vi "ultrasonic.vi"(0 "Ultrasonic configuration":string="{\n  \"type\": \"Ultrasonic\",\n  \"listen_port\": 8900,\n  \"location\": {\n    \"x\": 245.0,\n    \"y\": 0.0,\n    \"z\": 60.0\n  },\n  \"rotation\": {\n    \"pitch\": 0.0,\n    \"yaw\": 0.0,\n    \"roll\": 0.0\n  },\n  \"fc\": 40000.0,\n  \"pwm_factor\": 2.5,\n  \"max_ultrasonic_returns\": 93,\n   \"sbr\": {\n   \"scan_distance\":4.0,\n   \"azimuth_fov\":30.0,\n   \"elevation_fov\": 0.50,\n    \"ray_division_y\": 5.0,\n    \"ray_division_z\": 5.0,\n    \"debug_frustum\": false,\n    \"debug_scan\": false,\n    \"debug_rescan\": false\n  }\n}", 2 "error in":errorcluster) -> (3 "Ultrasonic Range":cluster{"targets":cluster{"range":dbl}[]}, 4 "Raw data":string, 5 "Ultrasonic configuration":string, 6 "error out":errorcluster)   [LabVIEW 2019]
doc: "Configures and samples the ultrasonic sensor according to the configuration settings. Provides range from the closest object to a single ultrasonic sensor."
uses:
  controls/Header.ctl
  tools/simx_common.vi
panel:
  out "Header":T1 {"game_time" format="%#_10g"}
  out "Ultrasonic Sensor Raw Data":string
  in  "ultrasonic_connection":refnum<k5>
  in  "null connection":refnum<k5>
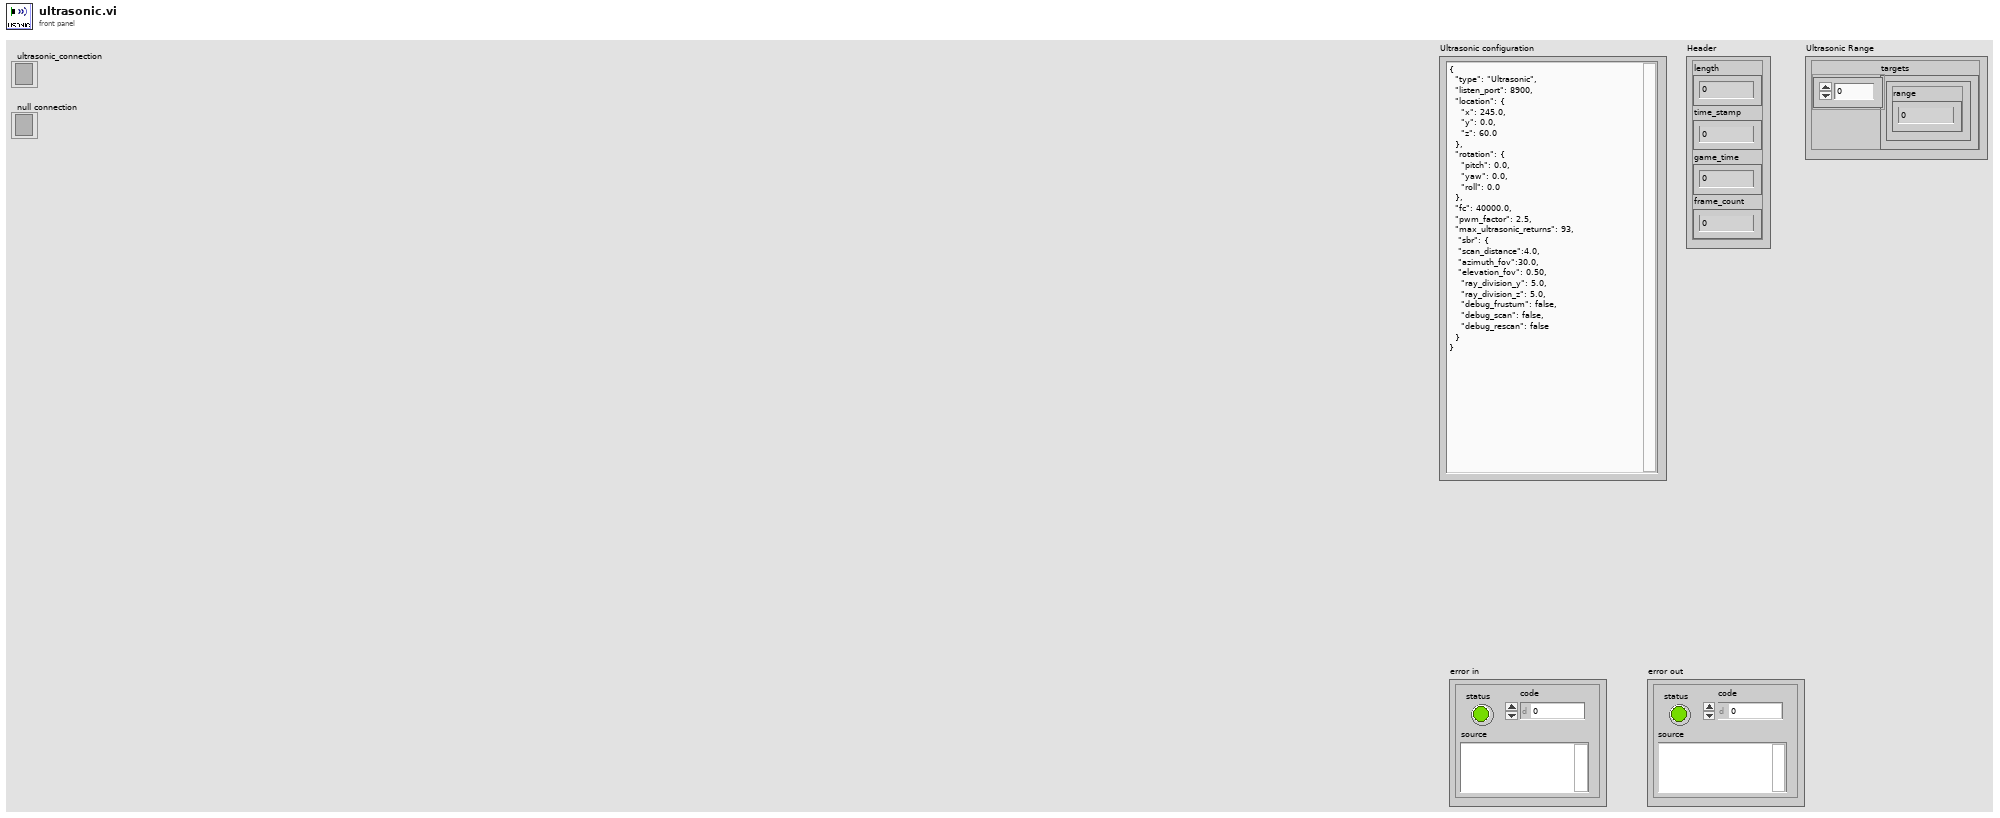
[diagram p1: front panel]
types:
  T1 = typedef "Header.ctl" = cluster{"length":u32, "time_stamp":u32, "game_time":sgl, "frame_count":u32}
  T2 = typedef "simx_connection.ctl" = cluster{"Config":T3, "Connections":T6, "Map":cluster{"lanes":cluster{"x":dbl[], "y":dbl[], "z":dbl[]}, "StartPosition":cluster{"start_points":T7, "StartRotation":dbl[], "StartLocation":dbl[]}, "Draw Map Size":T8, "DrawArea":cluster{"min_Y":dbl, "min_X":dbl, "Scale X":dbl, "Scale Y":dbl}, "Map":picture, "Map Geojson":string}}
  T3 = typedef "config.ctl" = cluster{"Trajectory":T4, "Weather":T5}
  T4 = typedef "trajectory.ctl" = cluster{"Number of frames":i32, "Frame number":i32, "Trajectory":string}
  T5 = typedef "weather.ctl" = cluster{"id":string}
  T6 = typedef "connections.ctl" = cluster{"Simulator Connection":refnum<k5>, "server_ip":string, "Port":i32, "Sensor connections":refnum<k5>[]}
  T7 = typedef "start_points.ctl" = cluster{"locations":dbl[][], "rotations":dbl[][], "type":string[]}
  T8 = typedef "LVBoundsTypeDef.ctl" = cluster{"Width":u32, "Height":u32}
  T9 = typedef "sensor_sample.ctl" = cluster{"Header":T1, "data out":string}
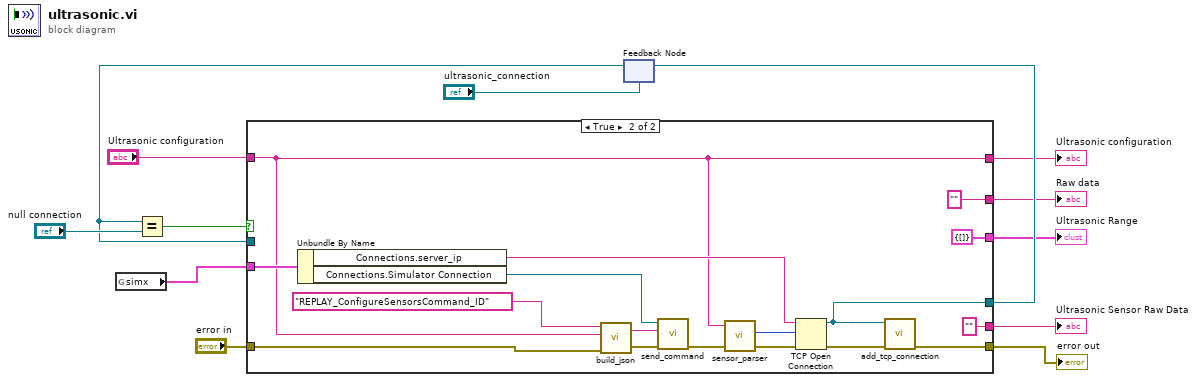
[diagram p0: block diagram]
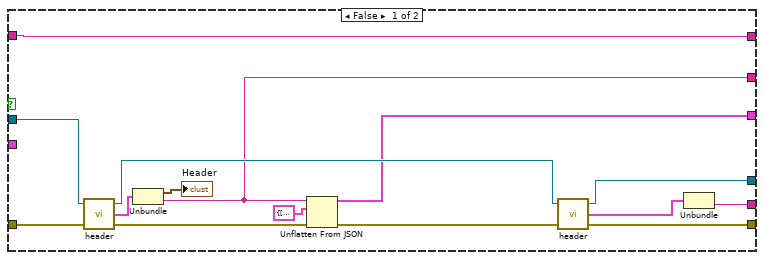
[diagram p2: hidden frame]
diagram:
  n1 = global read "simx_common.vi" "simx"() -> (w2:T2)
  n2 = feedback #1("ultrasonic_connection") -> (w7:refnum<k5>)
  n3 = Equal?(x=w7, y="null connection") -> (x = y?=w9:bool)
  n4 = case shown="True" w9 {
    tunnel: [w23 w34] -> w13
    tunnel: "Ultrasonic configuration" -> [w20 w30]
    tunnel: [w21 w33] -> w10
    tunnel: w7 -> [w27 _]
    tunnel: "error in" -> [w26 w40]
    tunnel: [w20 w30] -> w5
    tunnel: [w18 cluster{"targets":cluster{"range":dbl}[]} {"targets"=[]} ("Ultrasonic Range")] -> w4
    tunnel: [w17 "" ("data out")] -> w3
    tunnel: w2 -> [_ w37]
    tunnel: [w14 "" ("data out")] -> w1
    frame False {
      n5 = call "header.vi"("error in"=w26, "TCP Network Connection in"=w27) -> ("error out"=w24:errorcluster, "Sensor sample"=w28:T9, "TCP Network Connection out"=w25:refnum<k5>)  [unwired: 1 in]
      n6 = Unbundle(w28) -> ("Header"=→"Header":T1, "data out"=w17:string)
      n7 = Unflatten From JSON(JSON string=w17, type and defaults=cluster{"targets":cluster{"range":dbl}[]} {"targets"=[{"range"=0.0}]} ("Ultrasonic Range 2"), error in (no error)=w24) -> (value=w18:cluster{"targets":cluster{"range":dbl}[]}, error out=w22:errorcluster)  [unwired: 4 in]
      n8 = call "header.vi"("error in"=w22, "TCP Network Connection in"=w25) -> ("error out"=w23:errorcluster, "Sensor sample"=w15:T9, "TCP Network Connection out"=w21:refnum<k5>)  [unwired: 1 in]
      n9 = Unbundle(w15) -> ("data out"=w14:string)  [unwired: 1 out]
    }
    frame True {
      n10 = Unbundle By Name(w37) -> ("Connections.server_ip"=w36:string, "Connections.Simulator Connection"=w32:refnum<k5>)
      n11 = call "build_json.vi"("error in"=w40, "Message"=w30, "Command_ID"="REPLAY_ConfigureSensorsCommand_ID") -> ("error out"=w43:errorcluster, "JSON Out"=w44:string)  [unwired: 1 in]
      n12 = call "send_command.vi"("error in"=w43, "JSON Command"=w44, "TCP Network Connection in"=w32) -> ("error out"=w42:errorcluster)  [unwired: 1 in, 3 out]
      n13 = call "sensor_parser.vi"("Sensor configuration"=w30, "error in"=w42) -> ("Port out"=w29:u16, "error out"=w35:errorcluster)  [unwired: 1 in, 2 out]
      n14 = TCP Open Connection(address=w36, remote port or service name=w29, error in (no error)=w35) -> (connection ID=w33:refnum<k5>, error out=w41:errorcluster)  [unwired: 2 in]
      n15 = call "add_tcp_connection.vi"("error in"=w41, "Sensor connection"=w33) -> ("error out"=w34:errorcluster)  [unwired: 5 in]
    }
  }
  "error out" <- w13
  "Ultrasonic Sensor Raw Data" <- w1
  "Ultrasonic configuration" <- w5
  "Ultrasonic Range" <- w4
  "Raw data" <- w3
  n16 = feedback-in #1(w10) -> ()
